vi "logout reset login.vi"(4 "error in (no error)":errorcluster, 6 "POST Data (\"\")":string, 7 "Connection Refnum":T1) -> (0 "error out":errorcluster, 2 "new POST":string, 3 "dup Connection Refnum":T1)   [LabVIEW 2011]
uses:
  Summitek EXT/ODBC/SQL Controls/Connection Refnum.ctl
  ITK EXT/utils/strutil.llb/Case Matching.ctl
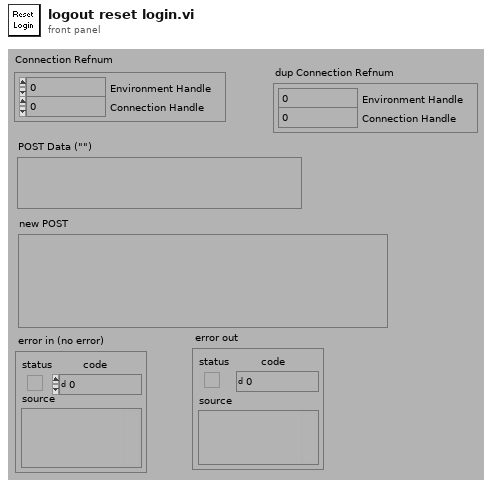
[diagram p1: front panel]
types:
  T1 = typedef "Connection Refnum.ctl" = cluster{"Environment Handle":i32, "Connection Handle":i32}
  T2 = typedef "Case Matching.ctl" = enum16{"a != A", "a == A", "system"}
  T3 = typedef "Keyed Array.ctl" = cluster{"keys":string[], "values":string[]}
  T4 = cluster{"To (\"\")":string, "From (\"\")":string, "Subject (\"\")":string, "HTMLBody (\"\")":string}
  T5 = typedef "User Record.ctl" = cluster{"ixUser":i32, "sxUsername":string, "sLastName":string, "sFirstName":string, "sEmail":string, "sPassword":string, "tLoginTime":timestamp, "sLoginComputer":string, "fAdministrator":bool, "fRunSequences":bool, "fModifySequences":bool, "fRunScenarios":bool, "fModifyScenarios":bool, "fModifyTemplates":bool, "fModifyUsers":bool, "fModifyStations":bool, "fModifyFields":bool}
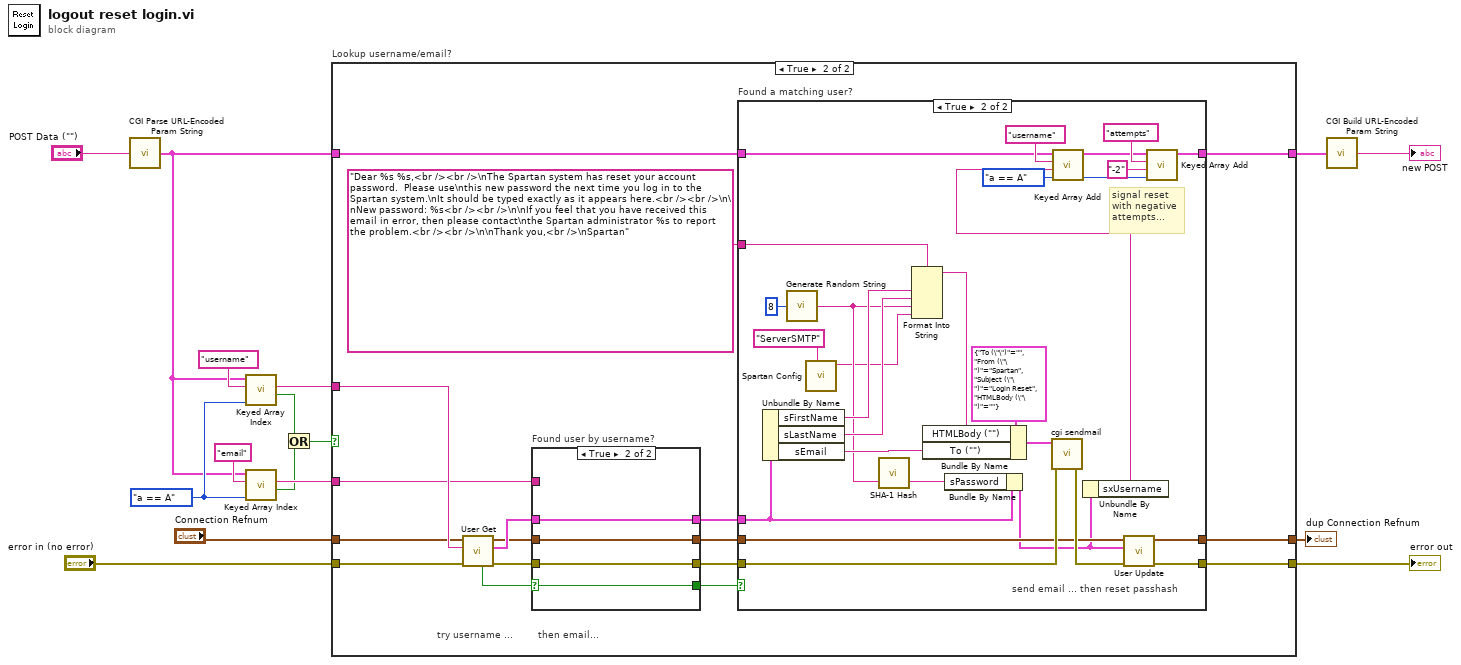
[diagram p0: block diagram]
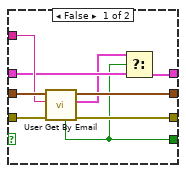
[diagram p4: hidden frame]
diagram:
  w14 = Case_Matching."a == A" ("case matching (sensitive)")
  n1 = call "CGI Parse URL-Encoded Param String.vi"("url-encoded param string"="POST Data (\"\")") -> ("params"=w5:T3)
  n2 = call "Keyed Array Index.vi"("case matching (sensitive)"=w14, "key"="username", "array in"=w5) -> ("valid key"=w8:bool, "value"=w12:string)  [unwired: 1 in, 2 out]
  n3 = call "Keyed Array Index.vi"("case matching (sensitive)"=w14, "key"="email", "array in"=w5) -> ("valid key"=w7:bool, "value"=w11:string)  [unwired: 1 in, 2 out]
  n4 = Or(x=w8, y=w7) -> (x .or. y?=w13:bool)
  n5 = case "Lookup username/email?" shown="True" w13 {
    tunnel: w12 -> [_ w28]
    tunnel: w11 -> [_ w27]
    tunnel: "error in (no error)" -> [w19 w23]
    tunnel: [w19 w21] -> w9
    tunnel: w5 -> [w18 w25]
    tunnel: [w18 w24] -> w4
    tunnel: "Connection Refnum" -> [w17 w22]
    tunnel: [w17 w20] -> w1
    frame False {
      # "Nothing to look up!"
    }
    frame True {
      # "then email..."
      # "try username ..."
      n6 = call "User Get.vi"("error in (no error)"=w23, "sxUsername (\"\")"=w28, "Connection Refnum"=w22) -> ("error out"=w35:errorcluster, "User"=w34:T5, "Connection Refnum"=w33:T1, "Data Present?"=w36:bool)  [unwired: 5 out]
      n7 = case "Found user by username?" shown="True" w36 {
        selector: w36 -> [_ w76]
        tunnel: w35 -> [w74 w77]
        tunnel: w34 -> [w70 w79]
        tunnel: w33 -> [w75 w78]
        tunnel: w27 -> [w73 _]
        tunnel: [w72 w77] -> w31
        tunnel: [w71 w78] -> w32
        tunnel: [w69 w79] -> w30
        tunnel: [w67 w76] -> w29
        frame False {
          n8 = call "User Get By Email.vi"("error in (no error)"=w74, "Email Address (\"\")"=w73, "Connection Refnum"=w75) -> ("error out"=w72:errorcluster, "User"=w68:T5, "Connection Refnum"=w71:T1, "Data Present?"=w67:bool)  [unwired: 5 out]
          n9 = Select(t=w68, s=w67, f=w70) -> (s? t:f=w69:T5)
        }
        frame True {
        }
      }
      n10 = case "Found a matching user?" shown="True" w29 {
        tunnel: w32 -> [w39 w63]
        tunnel: w31 -> [w38 w65]
        tunnel: [w39 w62] -> w20
        tunnel: w30 -> [_ w60]
        tunnel: [w38 w61] -> w21
        tunnel: "Dear %s %s,<br /><br />\nThe Spartan system has reset your account password.  Please use\nthis new password the next time you log in to the Spartan system.\nIt should be typed exactly as it appears here.<br /><br />\n\nNew password: %s<br /><br />\n\nIf you feel that you have received this email in error, then please contact\nthe Spartan administrator %s to report the problem.<br /><br />\n\nThank you,<br />\nSpartan" ("Subject (\"\")") -> [_ w56]
        tunnel: w25 -> [w37 w47]
        tunnel: [w37 w45] -> w24
        frame False {
        }
        frame True {
          w44 = Case_Matching."a == A" ("case matching (sensitive)")
          # "signal reset\nwith negative\nattempts..."
          # "send email ... then reset passhash"
          n11 = Unbundle By Name(w60) -> ("sFirstName"=w55:string, "sLastName"=w54:string, "sEmail"=w53:string)
          n12 = call "Generate Random String.vi"("String Length (5)"=8) -> ("Output String"=w52:string)  [unwired: 4 out]
          n13 = call "Spartan Config.vi"("Config Key (\"\")"="ServerSMTP") -> ("Config Value"=w40:string)  [unwired: 8 in, 2 out]
          n14 = call "SHA-1 Hash.vi"("Message (\"\")"=w52) -> ("SHA-1 Hash"=w51:string)  [unwired: 2 out]
          n15 = Format Into String(format string=w56, w55, w54, w52, w40) -> (resulting string=w57:string)  [unwired: 2 in, 1 out]
          n16 = Bundle By Name(cluster=T4 {"To (\"\")"="", "From (\"\")"="Spartan", "Subject (\"\")"="Login Reset", "HTMLBody (\"\")"=""} ("Email Details"), "HTMLBody (\"\")"=w57, "To (\"\")"=w53) -> (w58:T4)
          n17 = Bundle By Name(cluster=w60, "sPassword"=w51) -> (w50:T5)
          n18 = call "cgi sendmail.vi"("error in (no error)"=w65, "Email Details"=w58) -> ("error out"=w64:errorcluster)  [unwired: 2 in, 4 out]
          n19 = Unbundle By Name(w50) -> ("sxUsername"=w43:string)
          n20 = call "Keyed Array Add.vi"("case matching (sensitive)"=w44, "value"=w43, "key"="username", "array in"=w47) -> ("array out"=w46:T3)  [unwired: 3 out]
          n21 = call "User Update.vi"("error in (no error)"=w64, "User Record"=w50, "Connection Refnum"=w63) -> ("error out"=w61:errorcluster, "dup Connection Refnum"=w62:T1)  [unwired: 7 out]
          n22 = call "Keyed Array Add.vi"("case matching (sensitive)"=w44, "value"="-2", "key"="attempts", "array in"=w46) -> ("array out"=w45:T3)  [unwired: 3 out]
        }
      }
    }
  }
  "error out" <- w9
  "dup Connection Refnum" <- w1
  n23 = call "CGI Build URL-Encoded Param String.vi"("params"=w4) -> ("url-encoded param string"=→"new POST":string)
